vi "Errors.vi"   [LabVIEW 2021, in "DSF Core.lvlib" / "Transfer Group.lvclass"]
uses:
  Transfer Group.lvclass
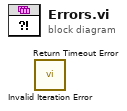
[diagram p0: block diagram]
diagram:
  n1 = call "Invalid Iteration Error.vi"() -> ()  [unwired: 10 in, 2 out]
  n2 = call "Return Timeout Error.vi"() -> ()  [unwired: 10 in, 2 out]
